vi "MGI AF Message Maker.vi"() -> ()   [LabVIEW 2015]
uses:
  Message Maker/Message Maker.lvclass
  Message Maker/Message Status.ctl
panel:
  in  "Project:":u16(ring) items=["AF Message Maker.lvproj"]
  in  "Actors":string[](tree)
  in  "Include Deps":bool caption="Include Actors in Dependencies?"
  in  "Update Outdated":bool
  in  "Build Messages":bool
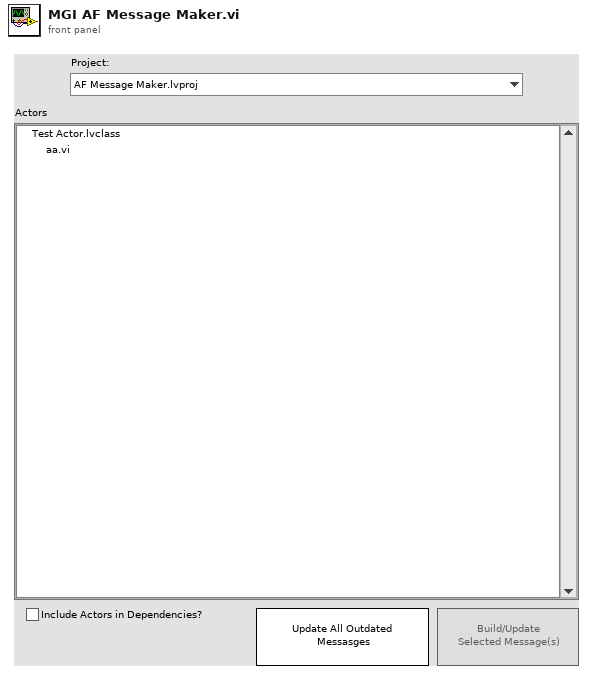
[diagram p1: front panel]
types:
  T1 = enum8{"Enabled", "Disabled", "Disabled and Grayed Out"}
  T2 = typedef "Message Maker.lvclass/Message Status.ctl" = enum16{"Message Not Created", "Message Out of Date", "Message OK", "Never update"}
  T3 = typedef "eventvkey.ctl" = enum16{"ASCII", "Enter", "Return", "Shift", "Ctrl", "Alt", "Cmd", "Opt", "Caps", "NumLock", "Clear", "Break", "Up", "Down", "Left", "Right", "Insert", "Delete", "Home", "End", "PageUp", "PageDown", "Escape", "Help", "Pause", "ScrollLock", "F1", "F2", "F3", "F4", "F5", "F6", "F7", "F8", "F9", "F10", "F11", "F12", "F13", "F14", "F15", "F16", "F17", "F18", "F19", "F20", "F21", "F22", "F23", "F24", "Play", "VolumeUp", "VolumeDown", "Mute", "Two Byte Char"}
  T4 = typedef "LVPoint32TypeDef.ctl" = cluster{"Horizontal":i32, "Vertical":i32}
  T5 = typedef "imagedata.ctl" = cluster{"image type":i32, "image depth":i32, "image":u8[], "mask":u8[], "colors":u32[], "Rectangle":cluster{"left":i16, "top":i16, "right":i16, "bottom":i16}}
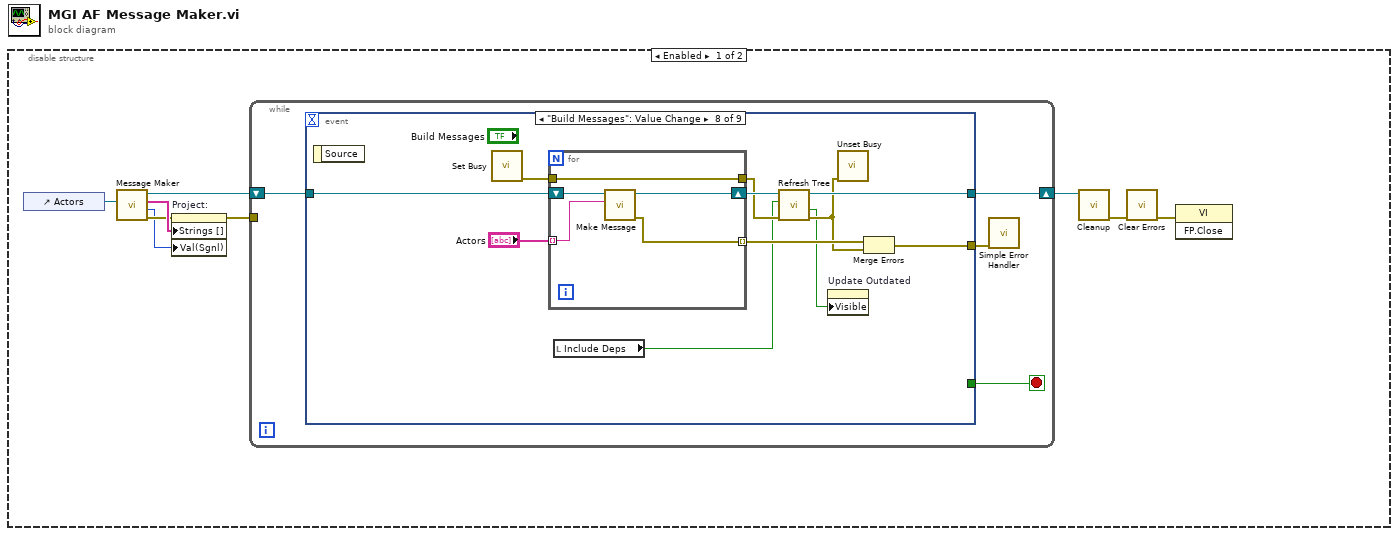
[diagram p0: block diagram]
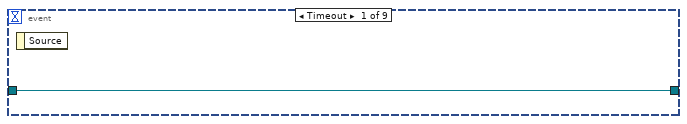
[diagram p2: hidden frame]
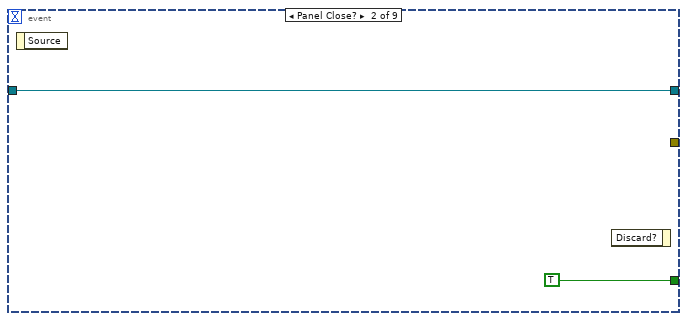
[diagram p3: hidden frame]
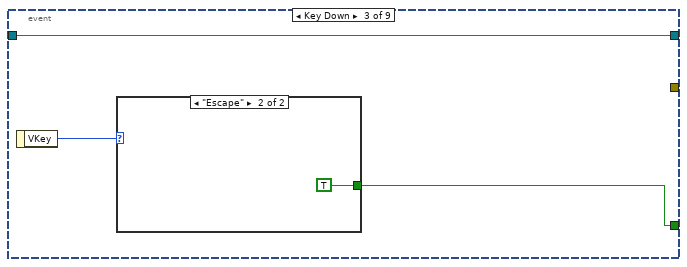
[diagram p4: hidden frame]
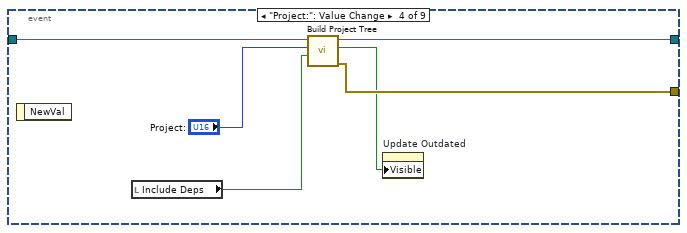
[diagram p6: hidden frame]
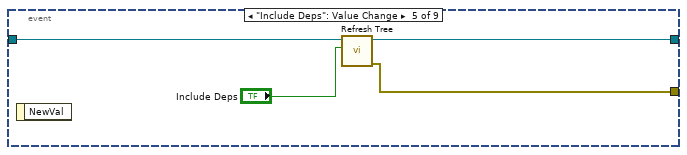
[diagram p7: hidden frame]
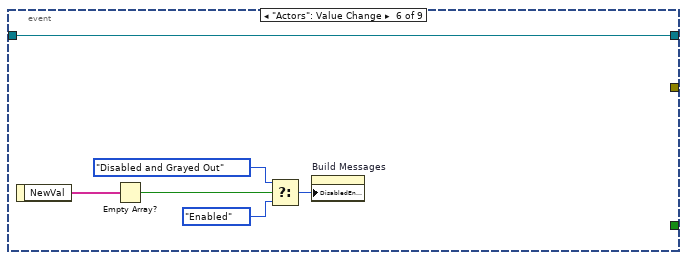
[diagram p8: hidden frame]
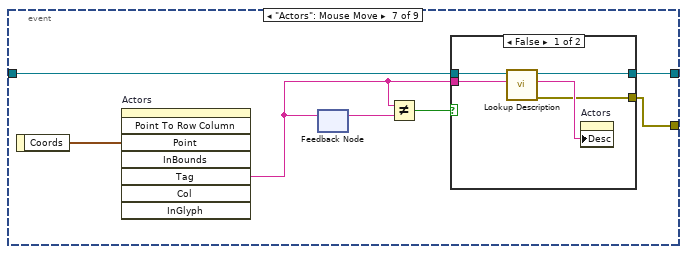
[diagram p9: hidden frame]
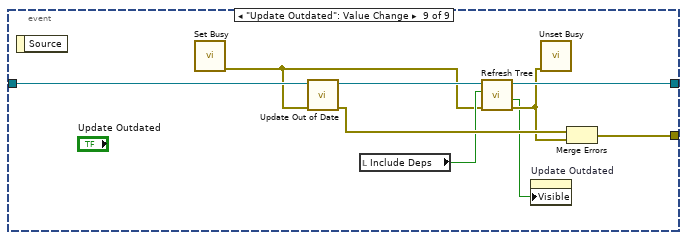
[diagram p11: hidden frame]
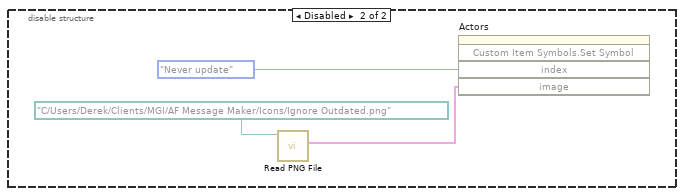
[diagram p12: hidden frame]
diagram:
  n1 = disable-structure shown="Enabled" {
    frame Enabled {
      n2 = control-ref of="Actors"() -> (w5:refnum<vi>)
      n3 = call "Message Maker.vi"("Actors Tree ref"=w5) -> ("error out"=w7:errorcluster, "Active Project"=w4:i32, "Projects"=w8:string[], "Message Maker out"=w9:refnum<class "Message Maker.lvclass">)  [unwired: 7 in]
      n4 = property on="Project:" class="Ring (strict)"(error in=w7, "Strings []"=w8, "Val(Sgnl)"=w4) -> (error out=w6:errorcluster)  [unwired: 1 in, 1 out]
      n5 = while {
        shift-right: [w12] -> w3
        shift-left: w9 -> [w13]
        tunnel: w6 -> [_]
        stop <- w11 stop-if-true
        n6 = event shown="[7] \"Build Messages\": Value Change" {
          selector: _ -> [_ _ _ _ _ _ _ _ _]
          dyn-events: _ -> [_ _ _ _ _ _ _ _ _]
          timeout: _ -> [_ _ _ _ _ _ _ _ _]
          tunnel: w13 -> [w14 w16 w19 w26 w30 w36 w42 w60 w74]
          tunnel: [w14 w16 w19 w25 w29 w36 w41 w56 w72] -> w12
          tunnel: [_ TRUE w17 _ _ _ _ _ _] -> w11
          tunnel: [_ _ _ w23 w27 _ w40 w53 w70] -> w10
          event Timeout {
            n7 = event-data() -> ()  [unwired: 1 in, 1 out]
          }
          event Panel Close? {
            n8 = event-data() -> ()  [unwired: 1 in, 1 out]
            n9 = event-data() -> ()  [unwired: 2 in, 1 out]
          }
          event Key Down {
            n10 = event-data() -> ("VKey"=w18:T3)  [unwired: 1 in]
            n11 = case shown="\"Escape\"" w18 {
              tunnel: [_ TRUE] -> w17
              frame "ASCII", Default {
              }
              frame "Escape" {
              }
            }
          }
          event "Project:": Value Change {
            n12 = event-data() -> ()  [unwired: 1 in, 1 out]
            n13 = local read "Include Deps"() -> (w22:bool)
            n14 = call "Build Project Tree.vi"("Include Dependencies?"=w22, "Project Index"="Project:", "Message Maker in"=w26) -> ("error out"=w23:errorcluster, "Messages out of Date?"=w21:bool, "Message Maker out"=w25:refnum<class "Message Maker.lvclass">)  [unwired: 6 in]
            n15 = property on="Update Outdated" class="Bool"("Visible"=w21) -> ()  [unwired: 2 in, 2 out]
          }
          event "Include Deps": Value Change {
            n16 = event-data() -> ()  [unwired: 1 in, 1 out]
            n17 = call "Refresh Tree.vi"("Include Dependencies?"="Include Deps", "Message Maker in"=w30) -> ("error out"=w27:errorcluster, "Message Maker out"=w29:refnum<class "Message Maker.lvclass">)  [unwired: 7 in, 1 out]
          }
          event "Actors": Value Change {
            n18 = event-data() -> ("NewVal"=w35:string[])  [unwired: 1 in]
            n19 = Empty Array?(array=w35) -> (empty?=w32:bool)
            n20 = Select(t=T1."Disabled and Grayed Out" ("Disabled"), s=w32, f=T1."Enabled" ("Disabled")) -> (s? t:f=w31:T1)
            n21 = property on="Build Messages" class="Bool"("DisabledEnum"=w31) -> ()  [unwired: 2 in, 2 out]
          }
          event "Actors": Mouse Move {
            n22 = event-data() -> ("Coords"=w43:T4)  [unwired: 1 in]
            n23 = invoke on="Actors" class="Tree (strict)" method="Point To Row Column"("Point"=w43) -> ("Tag"=w38:string)  [unwired: 7 in, 7 out]
            n24 = feedback-in #1(w38) -> ()
            n25 = feedback #1() -> (w37:string)  [unwired: 1 in]
            n26 = Not Equal?(x=w38, y=w37) -> (x != y?=w39:bool)
            n27 = case shown="False" w39 {
              tunnel: w42 -> [w48 w49]
              tunnel: [w47 w49] -> w41
              tunnel: w38 -> [w46 _]
              tunnel: [w44 _] -> w40
              frame False {
                n28 = call "Lookup Description.vi"("Tree Tag"=w46, "Message Maker in"=w48) -> ("error out"=w44:errorcluster, "Description"=w45:string, "Message Maker out"=w47:refnum<class "Message Maker.lvclass">)  [unwired: 7 in]
                n29 = property on="Actors" class="Tree (strict)"("Desc"=w45) -> ()  [unwired: 2 in, 2 out]
              }
              frame True {
              }
            }
          }
          event "Build Messages": Value Change {
            n30 = event-data() -> ()  [unwired: 1 in, 1 out]
            n31 = call <vilib>:"Set Busy.vi"() -> ("error out"=w58:errorcluster)  [unwired: 10 in, 1 out]
            n32 = for {
              shift-right: [w64] -> w57
              shift-left: w60 -> [w65]
              tunnel: "Actors" -> [w63] mode=indexing
              tunnel: w58 -> [w62]
              tunnel: [w62] -> w55
              tunnel: [w61] -> w54 mode=indexing
              n33 = call "Make Message.vi"("Method Qualified Name"=w63, "Message Maker in"=w65) -> ("error out"=w61:errorcluster, "Message Maker out"=w64:refnum<class "Message Maker.lvclass">)  [unwired: 8 in]
            }
            n34 = local read "Include Deps"() -> (w52:bool)
            n35 = call "Refresh Tree.vi"("error in (no error)"=w55, "Include Dependencies?"=w52, "Message Maker in"=w57) -> ("error out"=w51:errorcluster, "Messages out of date?"=w50:bool, "Message Maker out"=w56:refnum<class "Message Maker.lvclass">)  [unwired: 6 in]
            n36 = property on="Update Outdated" class="Bool"("Visible"=w50) -> ()  [unwired: 2 in, 2 out]
            n37 = call <vilib>:"Unset Busy.vi"("error in (no error)"=w51) -> ()  [unwired: 10 in, 1 out]
            n38 = Merge Errors(w54, w51) -> (w53:errorcluster)
          }
          event "Update Outdated": Value Change {
            n39 = event-data() -> ()  [unwired: 1 in, 1 out]
            n40 = call <vilib>:"Set Busy.vi"() -> ("error out"=w66:errorcluster)  [unwired: 10 in, 1 out]
            n41 = call "Update Out of Date.vi"("error in (no error)"=w66, "Message Maker in"=w74) -> ("error out"=w71:errorcluster, "Message Maker out"=w73:refnum<class "Message Maker.lvclass">)  [unwired: 8 in]
            n42 = local read "Include Deps"() -> (w69:bool)
            n43 = call "Refresh Tree.vi"("error in (no error)"=w66, "Include Dependencies?"=w69, "Message Maker in"=w73) -> ("error out"=w68:errorcluster, "Messages out of date?"=w67:bool, "Message Maker out"=w72:refnum<class "Message Maker.lvclass">)  [unwired: 6 in]
            n44 = property on="Update Outdated" class="Bool"("Visible"=w67) -> ()  [unwired: 2 in, 2 out]
            n45 = call <vilib>:"Unset Busy.vi"("error in (no error)"=w68) -> ()  [unwired: 10 in, 1 out]
            n46 = Merge Errors(w71, w68) -> (w70:errorcluster)
          }
        }
        n47 = call <vilib>:"Simple Error Handler.vi"("error in (no error)"=w10) -> ()  [unwired: 4 in, 5 out]
      }
      n48 = call "Cleanup.vi"("Message Maker in"=w3) -> ("error out"=w2:errorcluster)  [unwired: 10 in]
      n49 = call <vilib>:"Clear Errors.vi"("error in (no error)"=w2) -> ("error out"=w1:errorcluster)  [unwired: 5 in, 1 out]
      n50 = invoke class="VI" method="FP.Close"(error in=w1) -> ()  [unwired: 2 in, 3 out]
    }
    frame Disabled {
      n51 = call <vilib>:"Read PNG File.vi"("path to PNG file"=path "C:/Users/Derek/Clients/MGI/AF Message Maker/Icons/Ignore Outdated.png") -> ("image data"=w75:T5)  [unwired: 8 in, 2 out]
      n52 = invoke on="Actors" class="Tree (strict)" method="Custom Item Symbols.Set Symbol"("index"=Message_Status."Never update" ("Enum"), "image"=w75) -> ()  [unwired: 3 in, 5 out]
    }
  }
